vi "init.vi"(8 "error in (no error)":errorcluster, 10 "MUX Settings":T1, 11 "ConfigureILCDOStrategy in":refnum<class "ConfigureILCDOStrategy.lvclass">) -> (0 "error out":errorcluster, 3 "ConfigureILCDOStrategy out":refnum<class "ConfigureILCDOStrategy.lvclass">)   [LabVIEW 2015, in "ConfigureILCDOStrategy.lvclass"]
uses:
  ConfigureILCDOStrategy.lvclass
  Typedefs/MUX Settings.ctl
  Typedefs/Digital Signal Level.ctl
  ConfigureILCDOStrategy.lvclass/ConfigureILCDOStrategy.ctl
  Typedefs/ILCBTTypedefs.lvlib
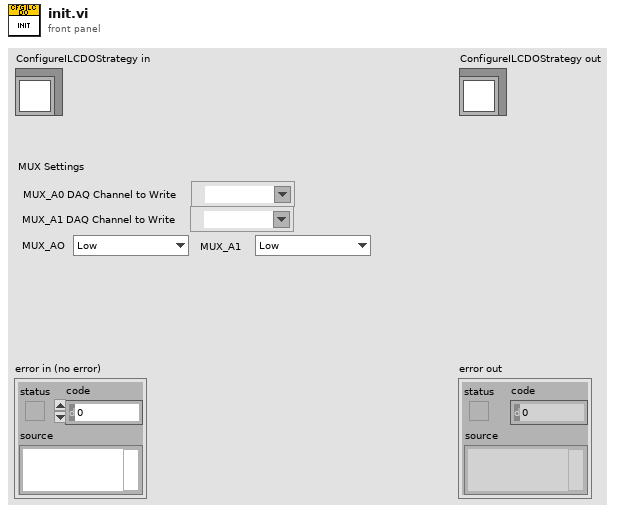
[diagram p1: front panel]
types:
  T1 = typedef "ILCBTTypedefs.lvlib/MUX Settings.ctl" = cluster{"MUX_AO":T2, "MUX_A1":T2, "MUX_A0 DAQ Channel to Write":refnum<k21>, "MUX_A1 DAQ Channel to Write":refnum<k21>}
  T2 = typedef "ILCBTTypedefs.lvlib/Digital Signal Level.ctl" = enum16{"Low", "High"}
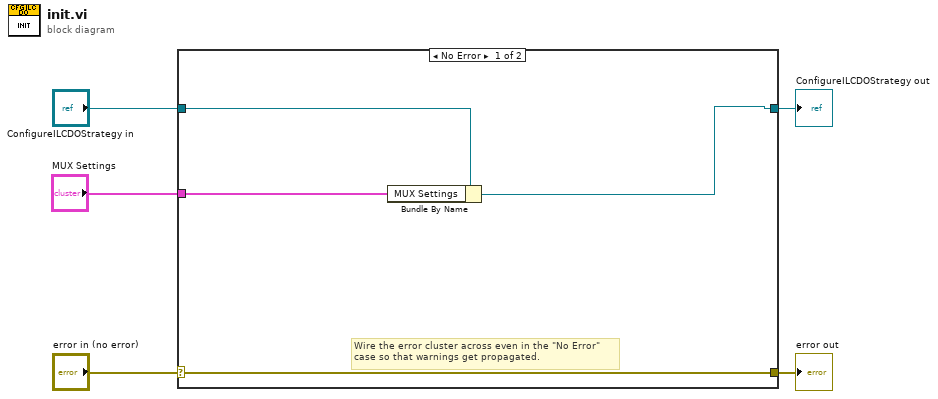
[diagram p0: block diagram]
diagram:
  n1 = case shown="No Error" "error in (no error)" {
    selector: "error in (no error)" -> [w9 w11]
    tunnel: [w9 w11] -> w4
    tunnel: [w7 w10] -> w2
    tunnel: "ConfigureILCDOStrategy in" -> [w8 w10]
    tunnel: "MUX Settings" -> [w6 _]
    frame No Error {
      # "Wire the error cluster across even in the \"No Error\"\ncase so that warnings get propagated."
      n2 = Bundle By Name(cluster=w8, "MUX Settings"=w6) -> (w7:refnum<class "ConfigureILCDOStrategy.lvclass">)
    }
    frame Error {
    }
  }
  "error out" <- w4
  "ConfigureILCDOStrategy out" <- w2
